vi "stepper motor Steps Counter.vi"() -> ()   [LabVIEW 2015]
panel:
  out "Numeric":i32
  in  "Stop":dbl=73.0 format="%#_13g"
  out "N":i32
  in  "Speed":dbl(slide)=100.0 scale=0.0..1000.0
  in  "States":bool[](array[boolean])
  in  "Start":dbl=73.0 format="%#_13g"
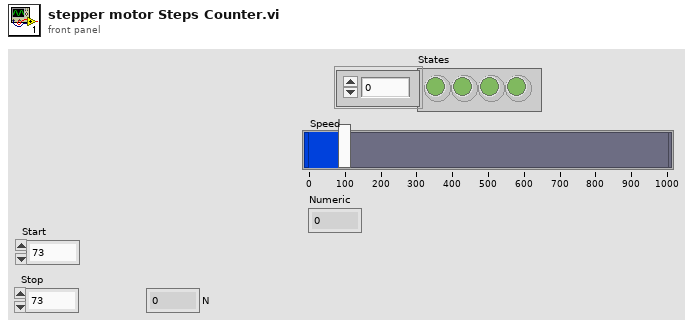
[diagram p1: front panel]
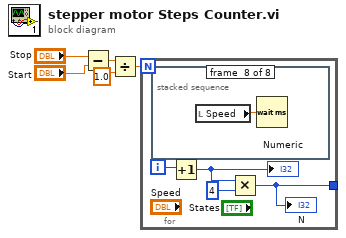
[diagram p0: block diagram]
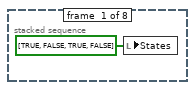
[diagram p2: hidden frame]
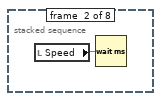
[diagram p3: hidden frame]
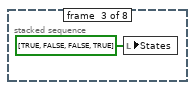
[diagram p4: hidden frame]
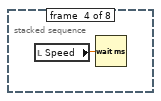
[diagram p5: hidden frame]
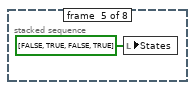
[diagram p6: hidden frame]
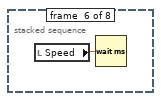
[diagram p7: hidden frame]
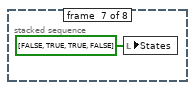
[diagram p8: hidden frame]
diagram:
  n1 = Subtract(x="Stop", y="Start") -> (x-y=w1:dbl)
  n2 = Divide(x=w1, y=1.0) -> (x/y=w5:dbl)
  n3 = for {
    N: w5 -> [_]
    tunnel: [w8] -> _
    i -> [w7]
    n4 = stacked-sequence {
      frame #0 {
        n5 = local write "States"(bool[] [TRUE, FALSE, TRUE, FALSE] ("Values")) -> ()
      }
      frame #1 {
        n6 = local read "Speed"() -> (w11:dbl)
        n7 = Wait (ms)(milliseconds to wait=w11) -> ()  [unwired: 1 out]
      }
      frame #2 {
        n8 = local write "States"(bool[] [TRUE, FALSE, FALSE, TRUE] ("Values")) -> ()
      }
      frame #3 {
        n9 = local read "Speed"() -> (w13:dbl)
        n10 = Wait (ms)(milliseconds to wait=w13) -> ()  [unwired: 1 out]
      }
      frame #4 {
        n11 = local write "States"(bool[] [FALSE, TRUE, FALSE, TRUE] ("Values")) -> ()
      }
      frame #5 {
        n12 = local read "Speed"() -> (w15:dbl)
        n13 = Wait (ms)(milliseconds to wait=w15) -> ()  [unwired: 1 out]
      }
      frame #6 {
        n14 = local write "States"(bool[] [FALSE, TRUE, TRUE, FALSE] ("Values")) -> ()
      }
      frame #7 {
        n15 = local read "Speed"() -> (w17:dbl)
        n16 = Wait (ms)(milliseconds to wait=w17) -> ()  [unwired: 1 out]
      }
    }
    n17 = Increment(x=w7) -> (x+1=w6:i32)
    "Numeric" <- w6
    n18 = Multiply(x=w6, y=4) -> (x*y=w8:i32)
    "N" <- w8
  }
